vi "StrMissingCount.vi"(8 "error in":errorcluster caption="错误输入（无错误）", 9 "BoolCtl":bool[](array[boolean]), 11 "IDStrIn":u32[](array[numeric])) -> (0 "error out":errorcluster caption="错误输出", 3 "StrOut":string)   [LabVIEW 2013]
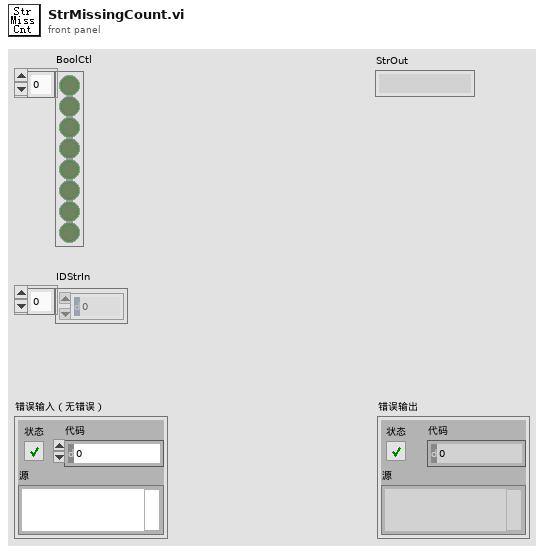
[diagram p1: front panel]
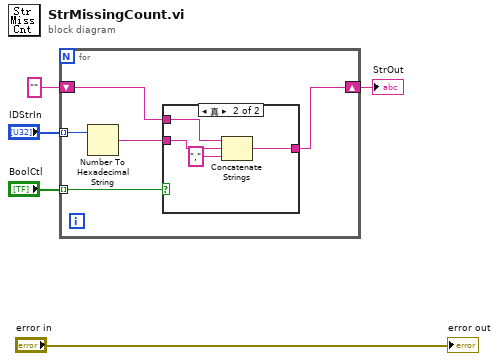
[diagram p0: block diagram]
diagram:
  n1 = for {
    shift-right: [w6] -> w2
    shift-left: "" -> [w7]
    tunnel: "IDStrIn" -> [w10] mode=indexing
    tunnel: "BoolCtl" -> [w9] mode=indexing
    n2 = Number To Hexadecimal String(2:w10) -> (0:w8:string)  [unwired: 1 in]
    n3 = case shown="真" w9 {
      tunnel: w8 -> [_ w14]
      tunnel: w7 -> [w11 w15]
      tunnel: [w11 w13] -> w6
      frame False {
      }
      frame True {
        n4 = Concatenate Strings(w15, w14, ",") -> (w13:string)
      }
    }
  }
  "StrOut" <- w2
  "error out" <- "error in"
